vi "Library Child VI URL.vi"(7 "Destination":path=path "", 8 "Error In":errorcluster, 11 "Name":string) -> (0 "Error Out":errorcluster, 3 "Child URL":string)   [LabVIEW 2018, in "Scripts.lvlib"]
uses:
  Scripts.lvlib
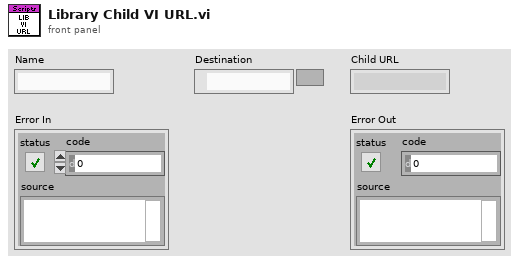
[diagram p1: front panel]
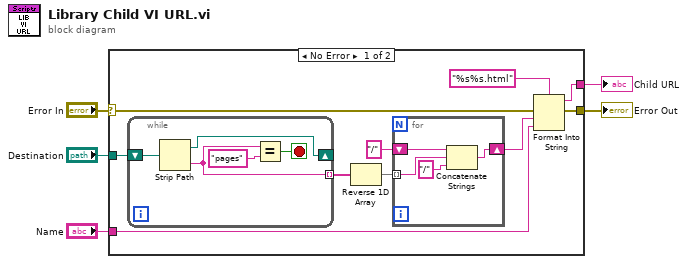
[diagram p0: block diagram]
diagram:
  n1 = case shown="No Error" "Error In" {
    selector: "Error In" -> [w6 w25]
    tunnel: "Name" -> [w14 _]
    tunnel: [w13 w25] -> w4
    tunnel: [w12 _] -> w3
    tunnel: "Destination" -> [w11 _]
    frame No Error {
      n2 = while {
        shift-right: [w22] -> _
        shift-left: w11 -> [w23]
        tunnel: [w20] -> w7 mode=indexing
        stop <- w21 stop-if-true
        n3 = Strip Path(path=w23) -> (stripped path=w22:path, name=w20:string)
        n4 = Equal?(x=w20, y="pages") -> (x = y?=w21:bool)
      }
      n5 = Reverse 1D Array(array=w7) -> (reversed array=w10:string[])
      n6 = for {
        tunnel: w10 -> [w18] mode=indexing
        shift-right: [w16] -> w8
        shift-left: "/" -> [w19]
        n7 = Concatenate Strings(w19, w18, "/") -> (w16:string)
      }
      n8 = Format Into String(format string="%s%s.html", error in=w6, w8, w14) -> (resulting string=w12:string, error out=w13:errorcluster)  [unwired: 1 in]
    }
    frame Error {
    }
  }
  "Error Out" <- w4
  "Child URL" <- w3
